vi "Create NI 9475 - Digital Output.vi"(8 "error in":errorcluster, 11 "channel settings":T1[](array[typedef])) -> (0 "error out":errorcluster, 3 "NI 9475 out":refnum<class "NI 9475.lvclass">)   [LabVIEW 2017, in "Scan Engine Scripting.lvlib" / "NI 9475.lvclass"]
uses:
  NI 9475.lvclass
  Mode Classes/Controls/digital channel settings.ctl
  Mode Classes/Digital Output Mode/Digital Output Mode.lvclass
  C:/dev/niveristand-scan-engine-ethercat-custom-device/Custom Device Source/Scripting/Modules/Mode Classes/Mode/Mode.lvclass
  d0f2271d-eb6b-4639-8b4f-5c6a815b042d.vi
  Scan Engine Scripting.lvlib
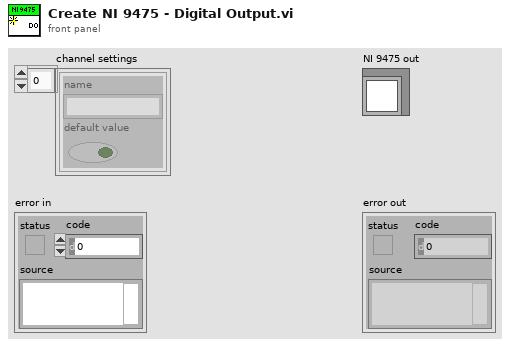
[diagram p1: front panel]
types:
  T1 = typedef "Scan Engine Scripting.lvlib/digital channel settings.ctl" = cluster{"name":string, "default value":bool}
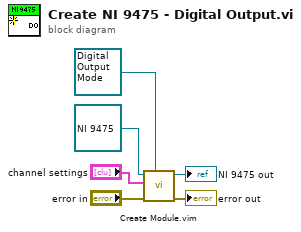
[diagram p0: block diagram]
diagram:
  n1 = call "Create Module.vim"("mode in"=refnum<class "Digital Output Mode.lvclass"> refnum ("Scan Engine Scripting.lvlib:Digital Output Mode.lvclass"), "error in"="error in", "channel settings"="channel settings", "module in"=refnum<class "NI 9475.lvclass"> refnum ("NI 9475 in")) -> ("error out"=→"error out":errorcluster, "module out"=→"NI 9475 out":refnum<class "NI 9475.lvclass">)  [unwired: 6 in]
